vi "Encode.vi"(8 "error in (no error)":errorcluster, 11 "ISO 14443 A UP in":refnum<class "ISO 14443 A UP.lvclass">) -> (0 "error out":errorcluster, 3 "ISO 14443 A UP out":refnum<class "ISO 14443 A UP.lvclass">)   [LabVIEW 2019, in "ISO 14443 A UP.lvclass"]
uses:
  ISO 14443 A UP.lvclass
  TypeDef/Store.ctl
  ISO 14443 A UP.lvclass/ISO 14443 A UP.ctl
  RFID system.lvclass
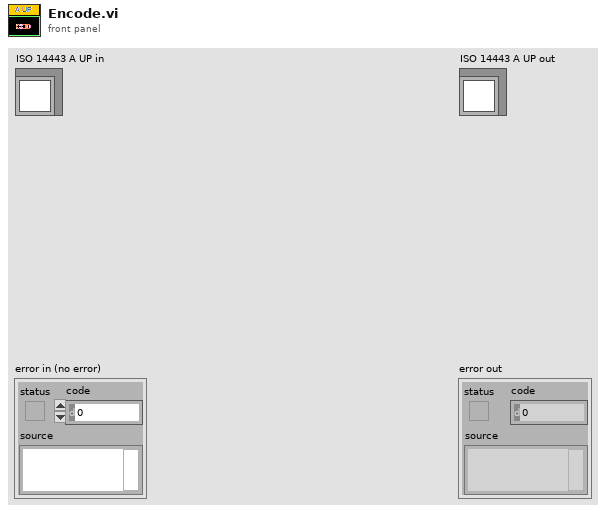
[diagram p1: front panel]
types:
  T1 = typedef "Store.ctl" = enum16{"envelope", "noise", "demSubCar", "CH_frame", "Decode", "demodulate", "in", "out", "sum", "subCarrier", "frame", "command", "encode", "modulate", "encode_UP", "modulate_up", "demod_up", "envelop_up", "sum_up", "out_up", "in_up"}
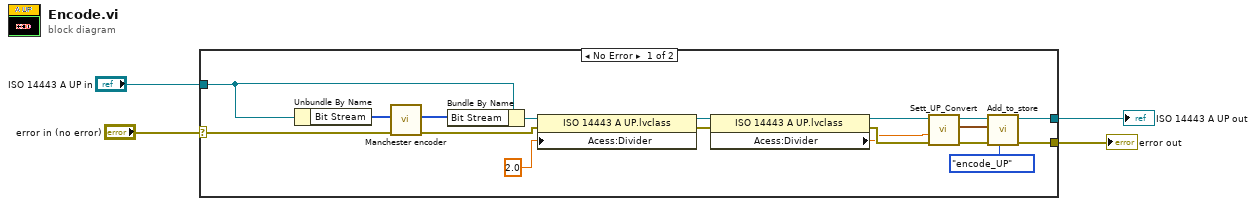
[diagram p0: block diagram]
diagram:
  n1 = case shown="No Error" "error in (no error)" {
    selector: "error in (no error)" -> [w14 w23]
    tunnel: "ISO 14443 A UP in" -> [w21 w24]
    tunnel: [w12 w24] -> w2
    tunnel: [w15 w23] -> w1
    frame No Error {
      n2 = Unbundle By Name(w21) -> ("Bit Stream"=w22:u8[])
      n3 = call "Manchester encoder.vi"("Error In"=w14, "Bit stream in"=w22) -> ("error out"=w8:errorcluster, "Bit stream out (Manchester encode)"=w20:u8[])  [unwired: 8 in]
      n4 = Bundle By Name(cluster=w21, "Bit Stream"=w20) -> (w19:refnum<class "ISO 14443 A UP.lvclass">)
      n5 = property class="ISO 14443 A UP.lvclass"(reference=w19, error in=w8, "Acess:Divider"=2.0 ("Divider(1)")) -> (reference out=w11:refnum<class "ISO 14443 A UP.lvclass">, error out=w7:errorcluster)
      n6 = property class="ISO 14443 A UP.lvclass"(reference=w11, error in=w7) -> (reference out=w10:refnum<class "ISO 14443 A UP.lvclass">, error out=w6:errorcluster, "Acess:Divider"=w5:dbl)
      n7 = call-dynamic "Sett_UP_Convert.vi"("error in (no error)"=w6, "Divider(1)"=w5, "ISO 14443 A UP in"=w10) -> ("error out"=w16:errorcluster, "Waveform"=w18:waveform(dbl), "ISO 14443 A UP out"=w17:refnum<class "ISO 14443 A UP.lvclass">)  [unwired: 6 in]
      n8 = call "Add_to_store.vi"("Store"=Store."encode_UP", "error in (no error)"=w16, "Waveform"=w18, "RFID system in"=w17) -> ("error out"=w15:errorcluster, "RFID system out"=w12:refnum<class "ISO 14443 A UP.lvclass">)  [unwired: 6 in]
    }
    frame Error {
    }
  }
  "error out" <- w1
  "ISO 14443 A UP out" <- w2
